vi "Load Sin Cos Files.vi"() -> (0 "Sin Fixed":fxp<+/-,32,1>[](array[numeric]), 1 "Sin Floating":dbl[](array[numeric]), 2 "Cos Fixed":fxp<+/-,32,1>[](array[numeric]), 3 "Cos Floating":dbl[](array[numeric]))   [LabVIEW 2015]
uses:
  <vilib>/Utility/file.llb/Read Delimited Spreadsheet (DBL).vi
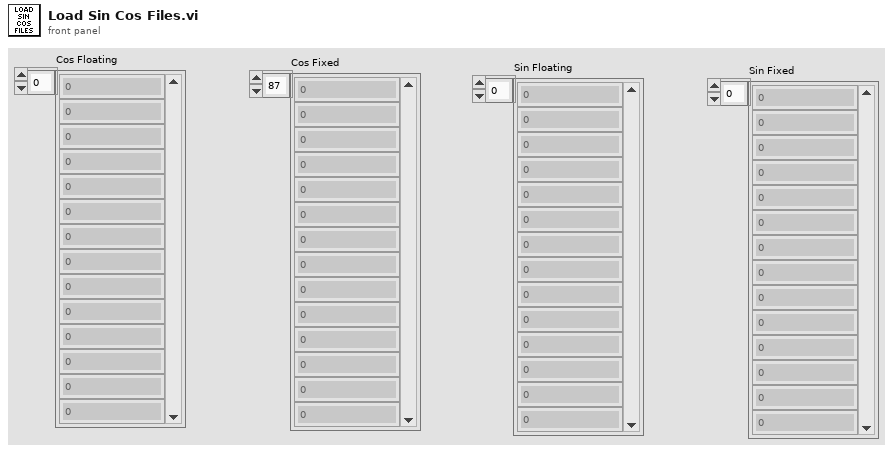
[diagram p1: front panel]
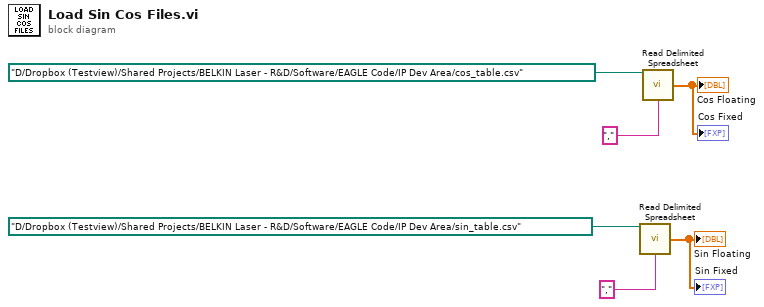
[diagram p0: block diagram]
diagram:
  n1 = call-poly <vilib>:"Read Delimited Spreadsheet.vi"("file path (dialog if empty)"=path "D:/Dropbox (Testview)/Shared Projects/BELKIN Laser - R&D/Software/EAGLE Code/IP Dev Area/sin_table.csv", "delimiter (\\t)"="," ("delimiter (\\t)")) -> ("first row"=→"Sin Floating" →"Sin Fixed":dbl[])  [unwired: 8 in, 5 out]
  n2 = call-poly <vilib>:"Read Delimited Spreadsheet.vi"("file path (dialog if empty)"=path "D:/Dropbox (Testview)/Shared Projects/BELKIN Laser - R&D/Software/EAGLE Code/IP Dev Area/cos_table.csv", "delimiter (\\t)"="," ("delimiter (\\t)")) -> ("first row"=→"Cos Floating" →"Cos Fixed":dbl[])  [unwired: 8 in, 5 out]
